vi "Read Thermometer Obj.vi"(11 "VacuumLines in":refnum<class "VacuumLines.lvclass">) -> (2 "Hardware.lvlib:Thermometer.lvlib:Thermometer.lvclass":refnum<class "Thermometer.lvclass">, 3 "VacuumLines out":refnum<class "VacuumLines.lvclass">)   [LabVIEW 2016, in "Hardware.lvlib" / "VacuumLine.lvlib" / "VacuumLines.lvclass"]
uses:
  <userlib>/Common Components/Hardware/Abstract System/VacuumLine/VacuumLines/VacuumLines.lvclass
  <userlib>/Common Components/Hardware/Thermometer/Thermometer.lvclass
  <userlib>/Common Components/Hardware/Abstract System/VacuumLine/VacuumLines/VacuumLines.lvclass/VacuumLines.ctl
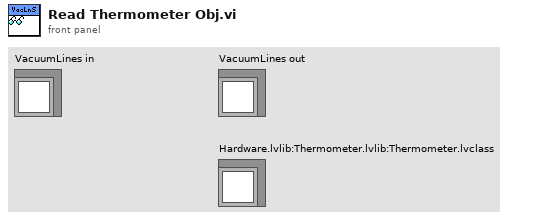
[diagram p1: front panel]
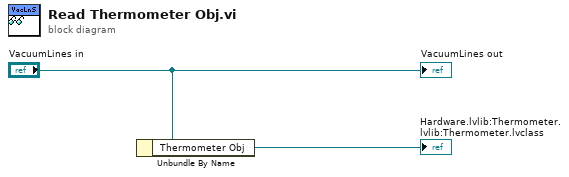
[diagram p0: block diagram]
diagram:
  n1 = Unbundle By Name("VacuumLines in") -> ("Thermometer Obj"=→"Hardware.lvlib:Thermometer.lvlib:Thermometer.lvclass":refnum<class "Thermometer.lvclass">)
  "VacuumLines out" <- "VacuumLines in"
